vi "ChannelRefresh.vi"(0 "Channel Setting 引用句柄":refnum<vi>) -> ()   [LabVIEW 2012]
panel:
  # "Channel 0 Settings"
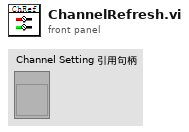
[diagram p1: front panel]
types:
  T1 = enum8{"Enabled", "Disabled", "Disabled and Grayed Out"}
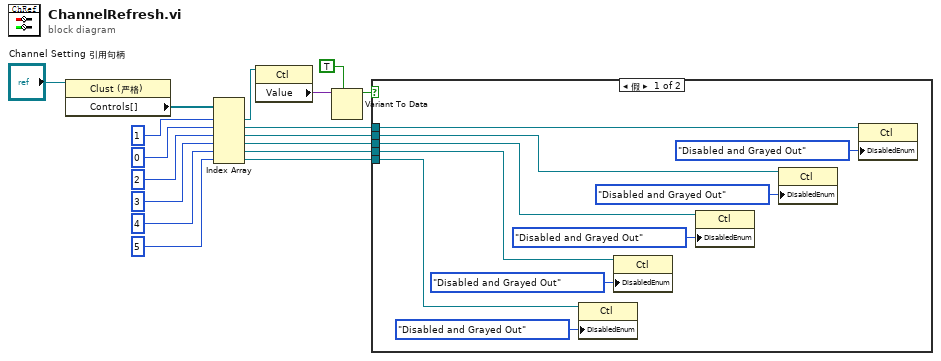
[diagram p0: block diagram]
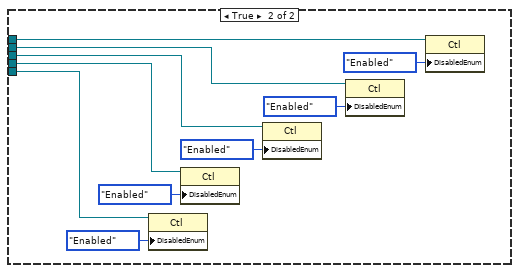
[diagram p2: hidden frame]
diagram:
  n1 = property class="Clust (严格)"(reference="Channel Setting 引用句柄") -> ("Controls[]"=w17:refnum<vi>[])  [unwired: 1 in, 2 out]
  n2 = Index Array(array=w17, index #1=1 ("索引"), index #2=0 ("索引"), index #3=2 ("索引"), index #4=3 ("索引"), index #5=4 ("索引"), index #6=5 ("索引")) -> (element #1=w15:refnum<vi>, element #2=w9:refnum<vi>, element #3=w8:refnum<vi>, element #4=w7:refnum<vi>, element #5=w6:refnum<vi>, element #6=w1:refnum<vi>)
  n3 = property class="Ctl"(reference=w15) -> ("Value"=w14:variant)  [unwired: 1 in, 2 out]
  n4 = Variant To Data(type=TRUE, Variant=w14) -> (data=w3:bool)  [unwired: 1 in, 1 out]
  n5 = case shown="假" w3 {
    tunnel: w9 -> [w23 w34]
    tunnel: w8 -> [w22 w31]
    tunnel: w7 -> [w21 w32]
    tunnel: w6 -> [w20 w33]
    tunnel: w1 -> [w19 w29]
    frame False {
      n6 = property class="Ctl"(reference=w19, "DisabledEnum"=T1."Disabled and Grayed Out" ("禁用")) -> ()  [unwired: 1 in, 2 out]
      n7 = property class="Ctl"(reference=w20, "DisabledEnum"=T1."Disabled and Grayed Out" ("禁用")) -> ()  [unwired: 1 in, 2 out]
      n8 = property class="Ctl"(reference=w21, "DisabledEnum"=T1."Disabled and Grayed Out" ("禁用")) -> ()  [unwired: 1 in, 2 out]
      n9 = property class="Ctl"(reference=w22, "DisabledEnum"=T1."Disabled and Grayed Out" ("禁用")) -> ()  [unwired: 1 in, 2 out]
      n10 = property class="Ctl"(reference=w23, "DisabledEnum"=T1."Disabled and Grayed Out" ("禁用")) -> ()  [unwired: 1 in, 2 out]
    }
    frame True {
      n11 = property class="Ctl"(reference=w29, "DisabledEnum"=T1."Enabled" ("禁用")) -> ()  [unwired: 1 in, 2 out]
      n12 = property class="Ctl"(reference=w33, "DisabledEnum"=T1."Enabled" ("禁用")) -> ()  [unwired: 1 in, 2 out]
      n13 = property class="Ctl"(reference=w32, "DisabledEnum"=T1."Enabled" ("禁用")) -> ()  [unwired: 1 in, 2 out]
      n14 = property class="Ctl"(reference=w31, "DisabledEnum"=T1."Enabled" ("禁用")) -> ()  [unwired: 1 in, 2 out]
      n15 = property class="Ctl"(reference=w34, "DisabledEnum"=T1."Enabled" ("禁用")) -> ()  [unwired: 1 in, 2 out]
    }
  }
